vi "decodeExt.vi"(8 "error in (no error)":errorcluster, 10 "ByteArray":u8[](array[numeric])) -> (0 "error out":errorcluster, 1 "BinaryArray":u8[](array[numeric]), 2 "variant":variant, 3 "RemainingBytes":u8[](array[numeric]), 5 "Type":string)   [LabVIEW 2020, in "MsgPack.lvlib"]
uses:
  MsgPack.lvlib
  <vilib>/Utility/error.llb/Error Cluster From Error Code.vi
  <vilib>/ErrorRing/Error Ring.xnode
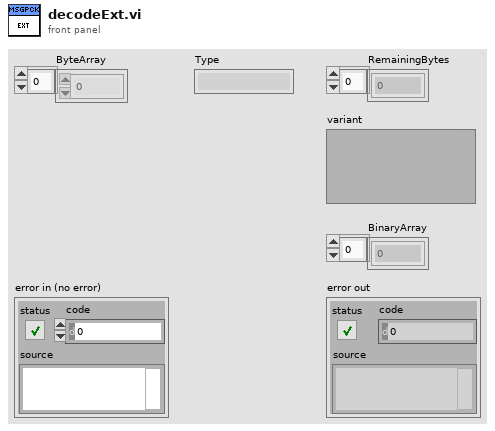
[diagram p1: front panel]
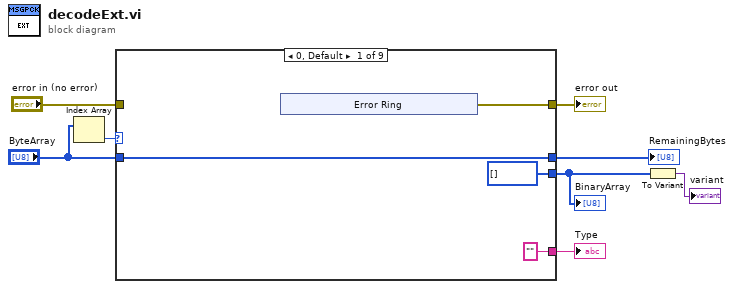
[diagram p0: block diagram]
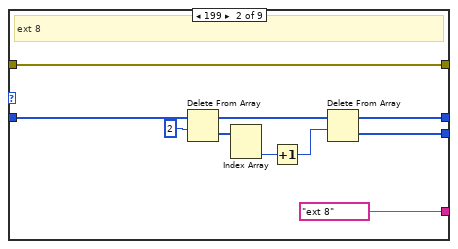
[diagram p2: hidden frame]
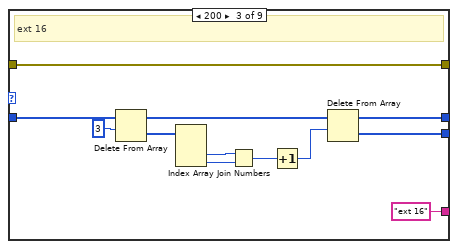
[diagram p3: hidden frame]
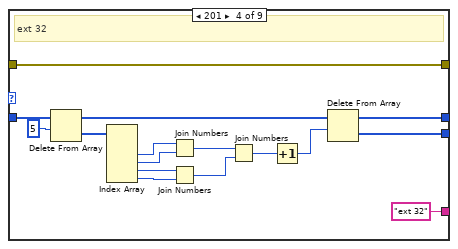
[diagram p4: hidden frame]
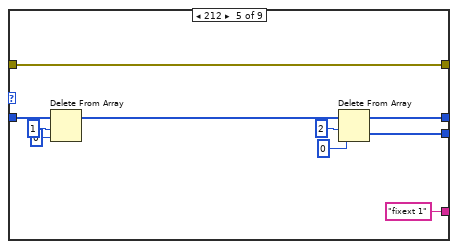
[diagram p5: hidden frame]
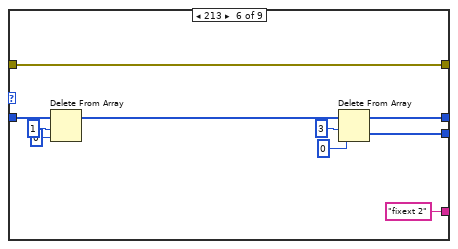
[diagram p6: hidden frame]
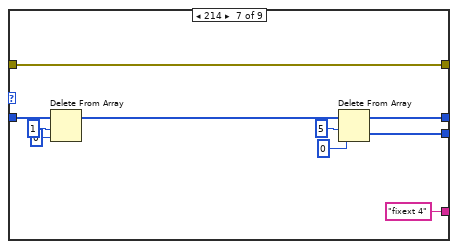
[diagram p7: hidden frame]
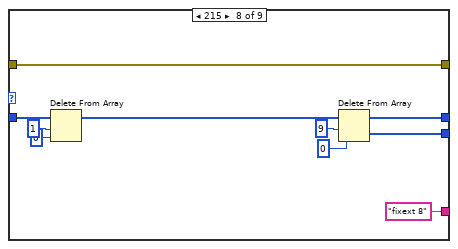
[diagram p8: hidden frame]
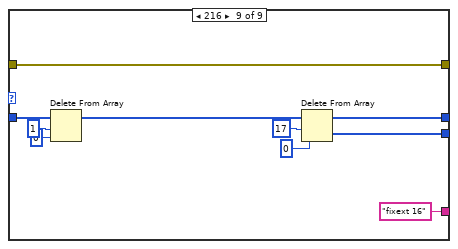
[diagram p9: hidden frame]
diagram:
  n1 = Index Array(array="ByteArray") -> (element=w5:u8)  [unwired: 1 in]
  n2 = case shown="0, Default" w5 {
    tunnel: [w11 w25 w38 w54 w65 w75 w85 w95 w105] -> w7
    tunnel: "error in (no error)" -> [_ w25 w38 w54 w65 w75 w85 w95 w105]
    tunnel: ["" "ext 8" "ext 16" "ext 32" "fixext 1" "fixext 2" "fixext 4" "fixext 8" "fixext 16"] -> w4
    tunnel: [u8[] [] w19 w29 w41 w58 w69 w78 w88 w98] -> w2
    tunnel: "ByteArray" -> [w9 w23 w33 w46 w63 w73 w80 w90 w100]
    tunnel: [w9 w18 w28 w40 w59 w68 w79 w89 w99] -> w1
    frame 0, Default {
      n3 = xnode "Error Ring"() -> ("error out"=w11:errorcluster)
    }
    frame 199 {
      # "ext 8"
      n4 = Delete From Array(array=w23, length=2 ("index")) -> (deleted portion=w22:u8[], array with subset deleted=w21:u8[])  [unwired: 1 in]
      n5 = Index Array(array=w22) -> (element #2=w26:u8)  [unwired: 2 in, 1 out]
      n6 = Increment(x=w26) -> (x+1=w20:u8)
      n7 = Delete From Array(array=w21, length=w20) -> (deleted portion=w19:u8[], array with subset deleted=w18:u8[])  [unwired: 1 in]
    }
    frame 200 {
      # "ext 16"
      n8 = Delete From Array(array=w33, length=u16 3 ("y")) -> (deleted portion=w32:u8[], array with subset deleted=w31:u8[])  [unwired: 1 in]
      n9 = Index Array(array=w32) -> (element #2=w36:u8, element #3=w37:u8)  [unwired: 3 in, 1 out]
      n10 = Join Numbers(hi=w36, lo=w37) -> ((hi.lo)=w35:u16)
      n11 = Increment(x=w35) -> (x+1=w30:u16)
      n12 = Delete From Array(array=w31, length=w30) -> (deleted portion=w29:u8[], array with subset deleted=w28:u8[])  [unwired: 1 in]
    }
    frame 201 {
      # "ext 32"
      n13 = Delete From Array(array=w46, length=u16 5 ("y")) -> (deleted portion=w44:u8[], array with subset deleted=w43:u8[])  [unwired: 1 in]
      n14 = Index Array(array=w44) -> (element #2=w52:u8, element #3=w53:u8, element #4=w51:u8, element #5=w50:u8)  [unwired: 5 in, 1 out]
      n15 = Join Numbers(hi=w52, lo=w53) -> ((hi.lo)=w48:u16)
      n16 = Join Numbers(hi=w51, lo=w50) -> ((hi.lo)=w49:u16)
      n17 = Join Numbers(hi=w48, lo=w49) -> ((hi.lo)=w47:u32)
      n18 = Increment(x=w47) -> (x+1=w42:u32)
      n19 = Delete From Array(array=w43, length=w42) -> (deleted portion=w41:u8[], array with subset deleted=w40:u8[])  [unwired: 1 in]
    }
    frame 212 {
      n20 = Delete From Array(array=w63, length=1, index=0) -> (array with subset deleted=w61:u8[])  [unwired: 1 out]
      n21 = Delete From Array(array=w61, length=u8 2 ("new element/subarray"), index=0) -> (deleted portion=w58:u8[], array with subset deleted=w59:u8[])
    }
    frame 213 {
      n22 = Delete From Array(array=w73, length=1, index=0) -> (array with subset deleted=w71:u8[])  [unwired: 1 out]
      n23 = Delete From Array(array=w71, length=u8 3 ("new element/subarray"), index=0) -> (deleted portion=w69:u8[], array with subset deleted=w68:u8[])
    }
    frame 214 {
      n24 = Delete From Array(array=w80, length=1, index=0) -> (array with subset deleted=w82:u8[])  [unwired: 1 out]
      n25 = Delete From Array(array=w82, length=u8 5 ("new element/subarray"), index=0) -> (deleted portion=w78:u8[], array with subset deleted=w79:u8[])
    }
    frame 215 {
      n26 = Delete From Array(array=w90, length=1, index=0) -> (array with subset deleted=w92:u8[])  [unwired: 1 out]
      n27 = Delete From Array(array=w92, length=u8 9 ("new element/subarray"), index=0) -> (deleted portion=w88:u8[], array with subset deleted=w89:u8[])
    }
    frame 216 {
      n28 = Delete From Array(array=w100, length=1, index=0) -> (array with subset deleted=w102:u8[])  [unwired: 1 out]
      n29 = Delete From Array(array=w102, length=u8 17 ("new element/subarray"), index=0) -> (deleted portion=w98:u8[], array with subset deleted=w99:u8[])
    }
  }
  "error out" <- w7
  "Type" <- w4
  "BinaryArray" <- w2
  "RemainingBytes" <- w1
  n30 = To Variant(anything=w2) -> (Variant=→"variant":variant)
